vi "PutPressureData.vi"(7 "shot":i32, 8 "Time":dbl[](array[numeric]), 9 "Pressure":dbl[](array[numeric]), 10 "Voltage":dbl[](array[numeric]), 11 "backup_directory":path) -> ()   [LabVIEW 2011]
panel:
  in  "Pressure Node Path":string="pressure:p2_ion_gauge:pressure"
  in  "Time Node Path":string="pressure:p2_ion_gauge:time"
  in  "Voltage Node Path":string="pressure:p2_ion_gauge:signal"
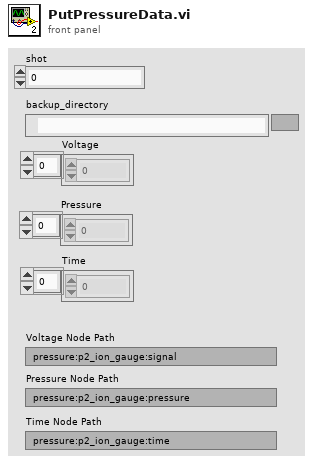
[diagram p1: front panel]
types:
  T1 = enum16{"open", "replace", "create", "open or create", "replace or create", "replace or create with confirmation"}
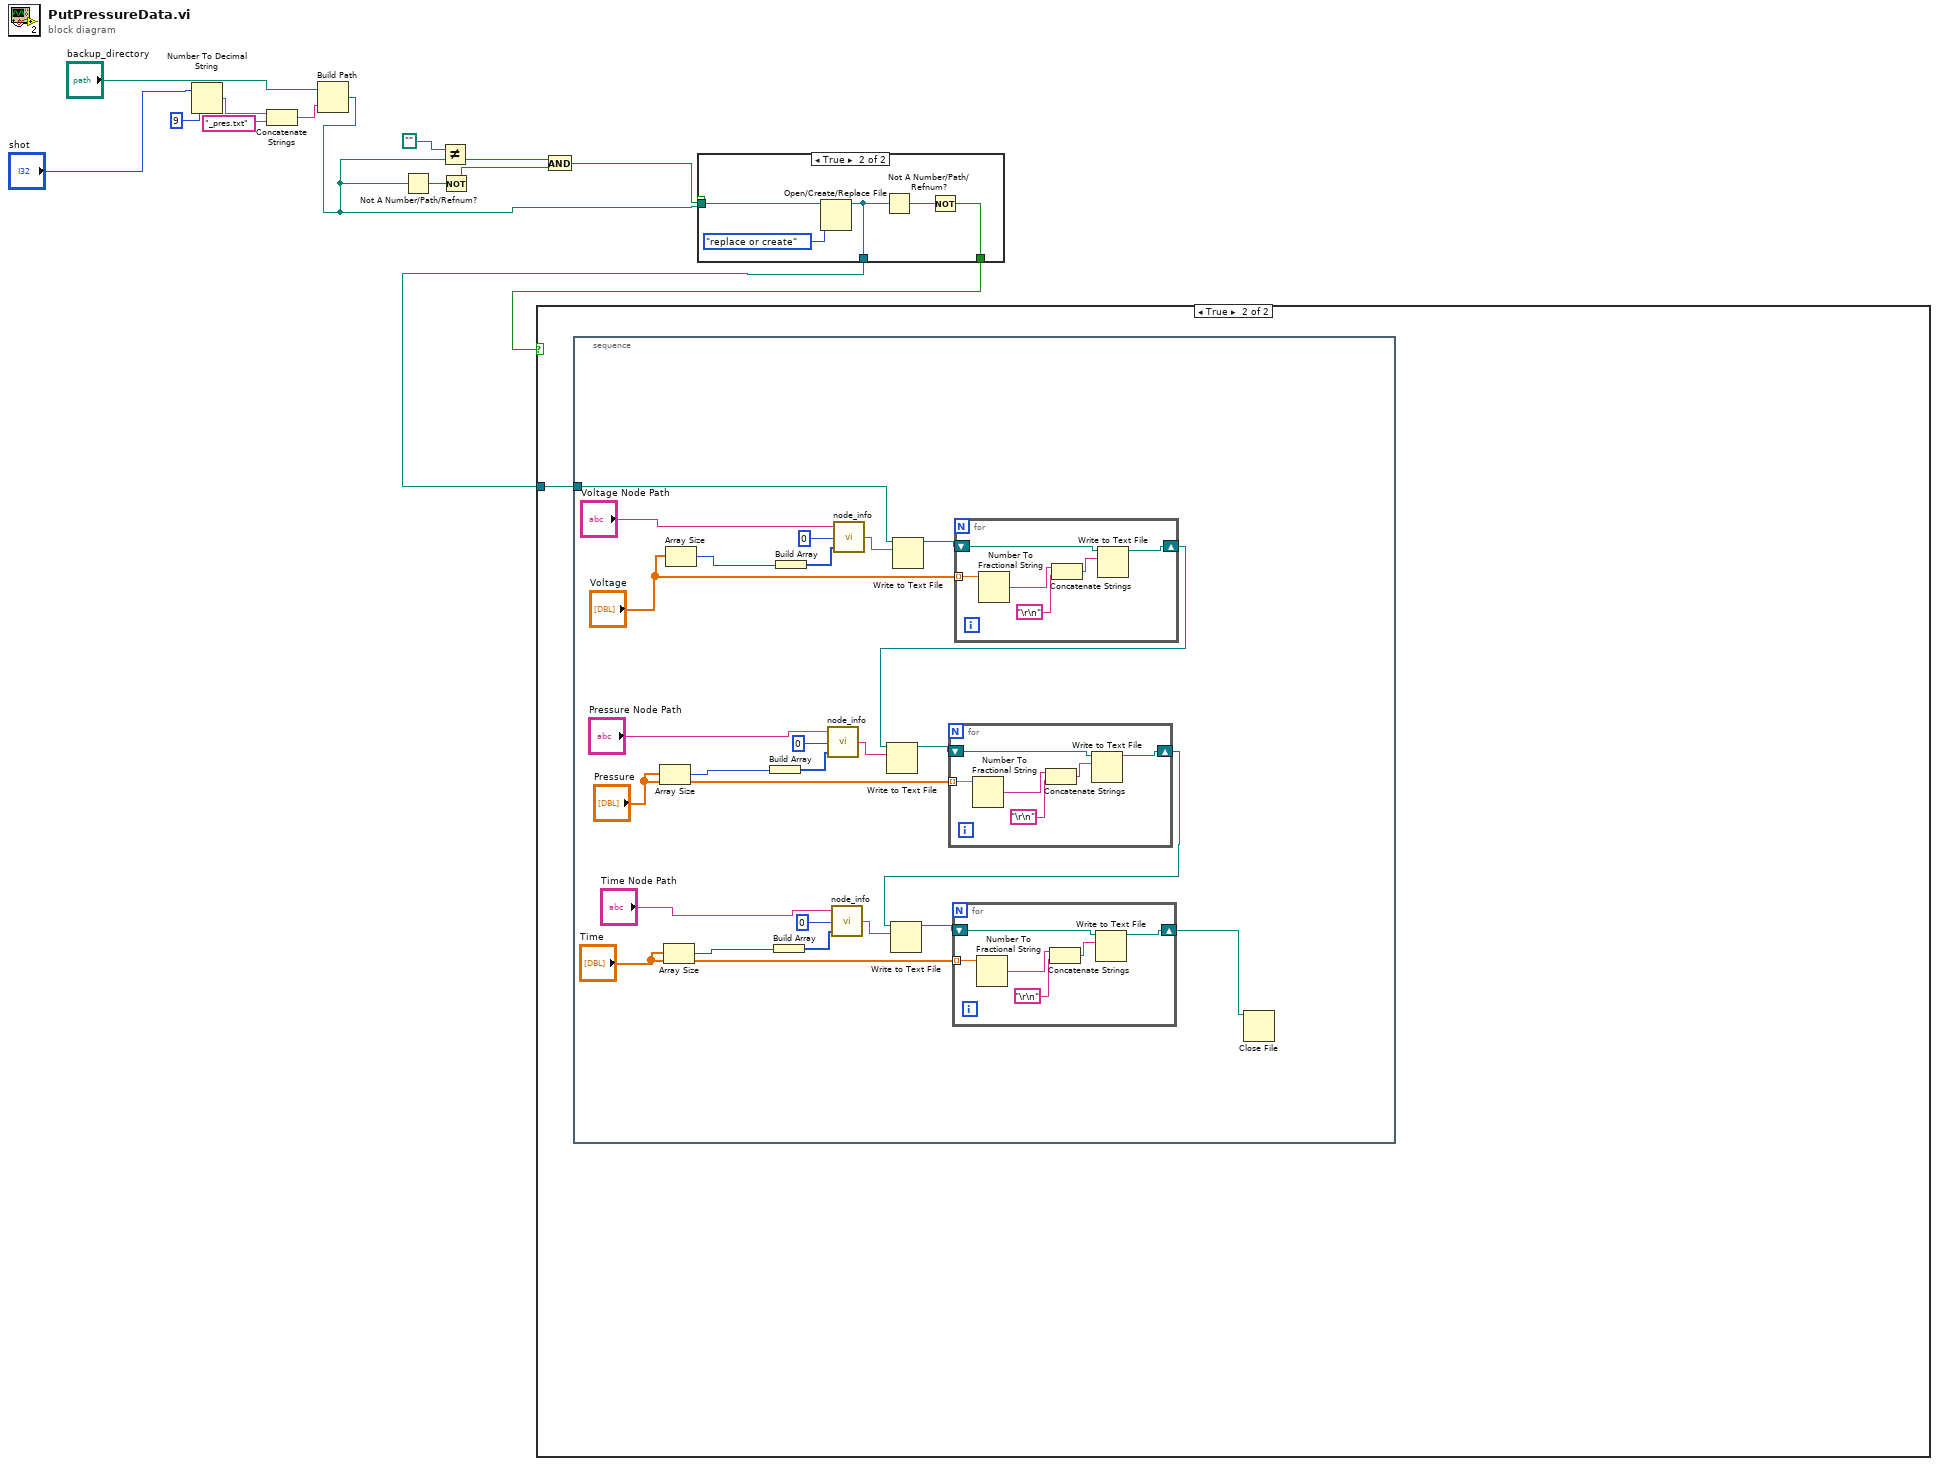
[diagram p0: block diagram]
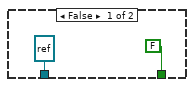
[diagram p3: hidden frame]
diagram:
  n1 = Number To Decimal String(number="shot", width (-)=i16 9) -> (decimal integer string=w7:string)
  n2 = Concatenate Strings(w7, "_pres.txt" ("string")) -> (w8:string)
  n3 = Build Path(base path="backup_directory", name or relative path=w8) -> (appended path=w5:path)
  n4 = Not A Number/Path/Refnum?(number/path/refnum=w5) -> (NaN/Path/Refnum?=w14:bool)
  n5 = Not Equal?(x=path "", y=w5) -> (x != y?=w12:bool)
  n6 = Not(x=w14) -> (.not. x?=w11:bool)
  n7 = And(x=w12, y=w11) -> (x .and. y?=w10:bool)
  n8 = case shown="True" w10 {
    tunnel: [FALSE w19] -> w2
    tunnel: [refnum<file> refnum ("refnum out") w18] -> w1
    tunnel: w5 -> [_ w17]
    frame False {
    }
    frame True {
      n9 = Open/Create/Replace File(file path (use dialog)=w17, operation (0:open)=T1."replace or create") -> (refnum out=w18:refnum<file>)  [unwired: 4 in, 2 out]
      n10 = Not A Number/Path/Refnum?(number/path/refnum=w18) -> (NaN/Path/Refnum?=w20:bool)
      n11 = Not(x=w20) -> (.not. x?=w19:bool)
    }
  }
  n12 = case shown="True" w2 {
    tunnel: w1 -> [_ w22]
    frame False {
    }
    frame True {
      n13 = stacked-sequence {
        tunnel: w22 -> [w42]
        frame #0 {
          n14 = Array Size(array="Pressure") -> (size(s)=w36:i32)
          n15 = Array Size(array="Time") -> (size(s)=w28:i32)
          n16 = Array Size(array="Voltage") -> (size(s)=w44:i32)
          n17 = Build Array(w36) -> (w37:i32[])
          n18 = Build Array(w28) -> (w29:i32[])
          n19 = Build Array(w44) -> (w45:i32[])
          n20 = call "node_info.vi"("Length"=w37, "Type"=0, "Name"="Pressure Node Path") -> ("Info"=w35:string)
          n21 = call "node_info.vi"("Length"=w29, "Type"=0, "Name"="Time Node Path") -> ("Info"=w27:string)
          n22 = call "node_info.vi"("Length"=w45, "Type"=0, "Name"="Voltage Node Path") -> ("Info"=w43:string)
          n23 = Write to Text File(file (use dialog)=w42, text=w43) -> (refnum out=w47:refnum<file>)  [unwired: 2 in, 2 out]
          n24 = for {
            shift-right: [w64] -> w34
            shift-left: w47 -> [w63]
            tunnel: "Voltage" -> [w60] mode=indexing
            n25 = Number To Fractional String(number=w60) -> (F-format string=w62:string)  [unwired: 3 in]
            n26 = Concatenate Strings(w62, "\r\n") -> (w65:string)
            n27 = Write to Text File(file (use dialog)=w63, text=w65) -> (refnum out=w64:refnum<file>)  [unwired: 2 in, 2 out]
          }
          n28 = Write to Text File(file (use dialog)=w34, text=w35) -> (refnum out=w39:refnum<file>)  [unwired: 2 in, 2 out]
          n29 = for {
            shift-right: [w58] -> w24
            shift-left: w39 -> [w57]
            tunnel: "Pressure" -> [w54] mode=indexing
            n30 = Number To Fractional String(number=w54) -> (F-format string=w56:string)  [unwired: 3 in]
            n31 = Concatenate Strings(w56, "\r\n") -> (w59:string)
            n32 = Write to Text File(file (use dialog)=w57, text=w59) -> (refnum out=w58:refnum<file>)  [unwired: 2 in, 2 out]
          }
          n33 = Write to Text File(file (use dialog)=w24, text=w27) -> (refnum out=w31:refnum<file>)  [unwired: 2 in, 2 out]
          n34 = for {
            shift-right: [w52] -> w23
            shift-left: w31 -> [w51]
            tunnel: "Time" -> [w48] mode=indexing
            n35 = Number To Fractional String(number=w48) -> (F-format string=w50:string)  [unwired: 3 in]
            n36 = Concatenate Strings(w50, "\r\n") -> (w53:string)
            n37 = Write to Text File(file (use dialog)=w51, text=w53) -> (refnum out=w52:refnum<file>)  [unwired: 2 in, 2 out]
          }
          n38 = Close File(refnum=w23) -> ()  [unwired: 1 in, 2 out]
        }
      }
    }
  }
